vi "Boiler Controller.vi"(8 "error in (no error)":errorcluster, 11 "Message Queues":T1) -> (0 "error out":errorcluster)   [LabVIEW 2015]
uses:
  support/Message Queue/All Message Queues.ctl
  support/Message Queue/Message Cluster.ctl
  support/Message Queue/Message Queue.lvlib
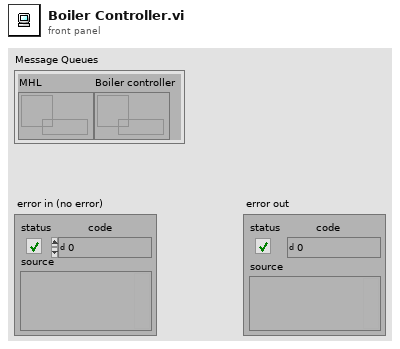
[diagram p1: front panel]
types:
  T1 = typedef "Message Queue.lvlib/All Message Queues.ctl" = cluster{"MHL":refnum<queue>, "Boiler controller":refnum<queue>}
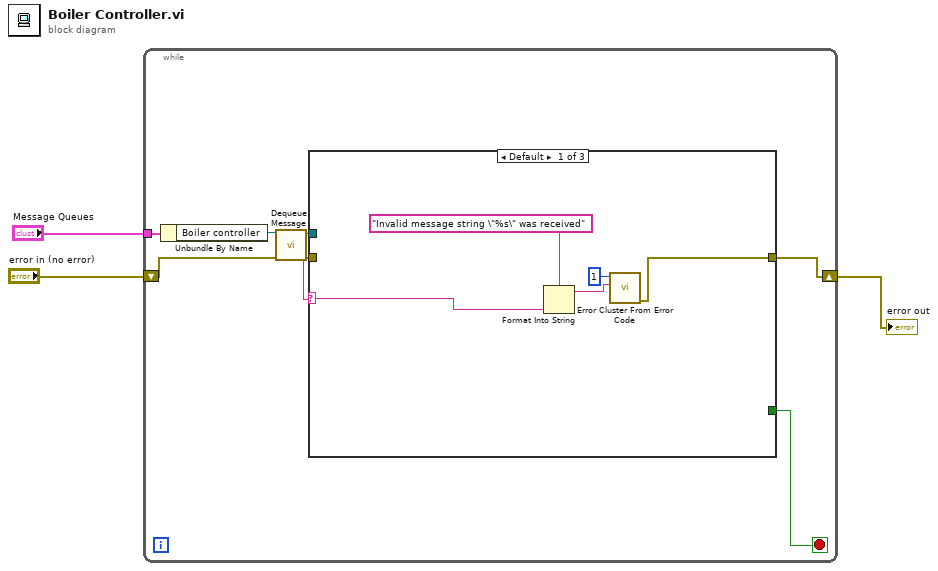
[diagram p0: block diagram]
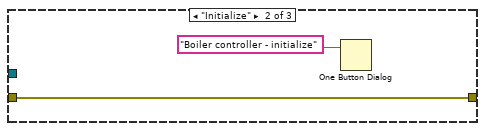
[diagram p2: hidden frame]
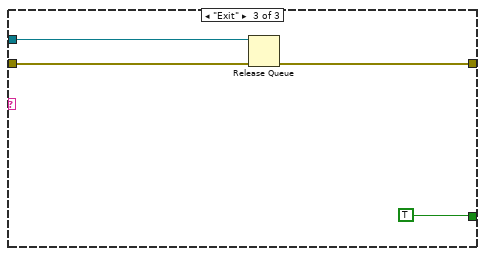
[diagram p3: hidden frame]
diagram:
  n1 = while {
    tunnel: "Message Queues" -> [w11]
    shift-right: [w5] -> w1
    shift-left: "error in (no error)" -> [w9]
    stop <- w4 stop-if-true
    n2 = Unbundle By Name(w11) -> ("Boiler controller"=w10:refnum<queue>)
    n3 = call "Dequeue Message.vi"("error in (no error)"=w9, "Message Queue"=w10) -> ("error out"=w7:errorcluster, "Message"=w6:string, "dup Message Queue"=w8:refnum<queue>)  [unwired: 6 in, 1 out]
    n4 = case shown="Default" w6 {
      selector: w6 -> [w16 _ _]
      tunnel: w8 -> [_ _ w20]
      tunnel: w7 -> [_ w18 w22]
      tunnel: [w12 w18 w21] -> w5
      tunnel: [_ _ TRUE] -> w4
      frame Default {
        n5 = Format Into String(format string="Invalid message string \"%s\" was received" ("initial string"), w16) -> (resulting string=w14:string)  [unwired: 2 in, 1 out]
        n6 = call <vilib>:"Error Cluster From Error Code.vi"("error message (\"\")"=w14, "error code (0)"=1) -> ("error out"=w12:errorcluster)  [unwired: 7 in]
      }
      frame "Initialize" {
        n7 = One Button Dialog(message="Boiler controller - initialize") -> ()  [unwired: 1 in, 1 out]
      }
      frame "Exit" {
        n8 = Release Queue(queue=w20, error in (no error)=w22) -> (error out=w21:errorcluster)  [unwired: 1 in, 2 out]
      }
    }
  }
  "error out" <- w1
